vi "Refresh ECUs.vi"(8 "Type (Input)":T1, 9 "Frame Index":u32, 10 "ECU Name":string, 11 "ECUs":T2[](array[typedef])) -> (3 "ECUs out":T2[](array[typedef]))   [LabVIEW 2020, in "Communication Bus Template System Explorer.lvlib" / "Implementation.lvlib"]
uses:
  Implementation.lvlib
  Types/ECU.ctl
  <vilib>/NI VeriStand/Custom Device API/Custom Device Channel Type.ctl
  <vilib>/NI VeriStand/Custom Device API/Custom Device API.lvlib
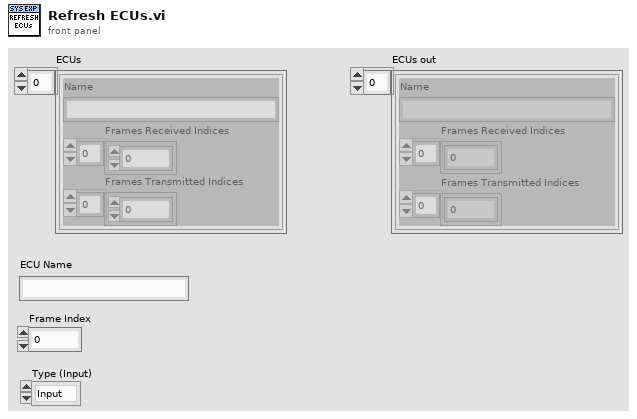
[diagram p1: front panel]
types:
  T1 = typedef "Custom Device API.lvlib/Custom Device Channel Type.ctl" = enum16{"Input", "Output"}
  T2 = typedef "Communication Bus Template System Explorer.lvlib/Implementation.lvlib/ECU.ctl" = cluster{"Name":string, "Frames Received Indices":u32[], "Frames Transmitted Indices":u32[]}
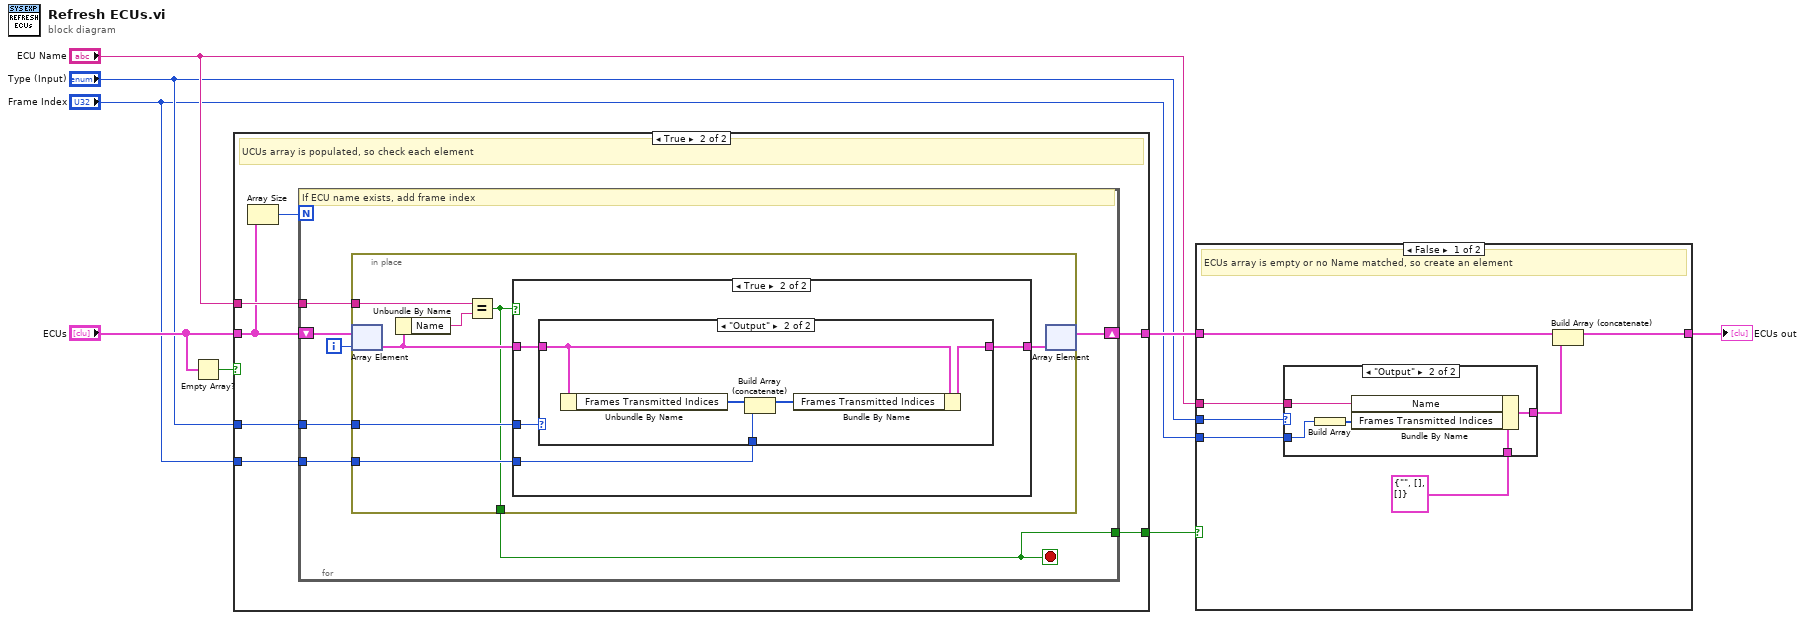
[diagram p0: block diagram]
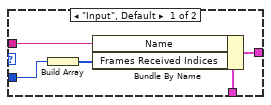
[diagram p2: hidden frame]
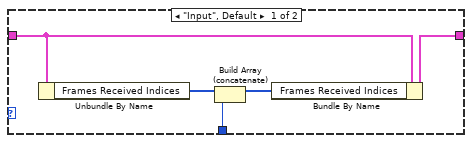
[diagram p6: hidden frame]
diagram:
  n1 = Empty Array?(array="ECUs") -> (empty?=w7:bool)
  n2 = case shown="True" w7 {
    selector: w7 -> [w9 _]
    tunnel: "ECU Name" -> [_ w17]
    tunnel: "Type (Input)" -> [_ w15]
    tunnel: "Frame Index" -> [_ w14]
    tunnel: [w10 w13] -> w5
    tunnel: "ECUs" -> [w10 w12]
    tunnel: [w9 w11] -> w6
    frame False {
      # "ECUs array is empty - need to create new element"
    }
    frame True {
      # "UCUs array is populated, so check each element"
      n3 = Array Size(array=w12) -> (size(s)=w16:i32)
      n4 = for {
        N: w16 -> [_]
        tunnel: w17 -> [w22]
        shift-right: [w19] -> w13
        shift-left: w12 -> [w24]
        tunnel: w15 -> [w21]
        tunnel: w14 -> [w20]
        tunnel: [w18] -> w11
        i -> [w23]
        stop <- w18 stop-if-true
        # "If ECU name exists, add frame index"
        n5 = in-place {
          in-place-border: w22 -> [w30]
          in-place-border: w21 -> [w28]
          in-place-border: w20 -> [w27]
          in-place-border: [w25] -> w18
          n6 = in-place-array #1(w24, w23) -> (w29:T2)
          n7 = Unbundle By Name(w29) -> ("Name"=w31:string)
          n8 = Equal?(x=w30, y=w31) -> (x = y?=w25:bool)
          n9 = case shown="True" w25 {
            tunnel: w29 -> [w32 w36]
            tunnel: w28 -> [_ w35]
            tunnel: w27 -> [_ w34]
            tunnel: [w32 w33] -> w26
            frame False {
            }
            frame True {
              n10 = case shown="\"Output\"" w35 {
                tunnel: w36 -> [w37 w42]
                tunnel: w34 -> [w40 w45]
                tunnel: [w38 w43] -> w33
                frame "Input", Default {
                  n11 = Unbundle By Name(w37) -> ("Frames Received Indices"=w41:u32[])
                  n12 = Build Array (concatenate)(w41, w40) -> (w39:u32[])
                  n13 = Bundle By Name(cluster=w37, "Frames Received Indices"=w39) -> (w38:T2)
                }
                frame "Output" {
                  n14 = Unbundle By Name(w42) -> ("Frames Transmitted Indices"=w46:u32[])
                  n15 = Build Array (concatenate)(w46, w45) -> (w44:u32[])
                  n16 = Bundle By Name(cluster=w42, "Frames Transmitted Indices"=w44) -> (w43:T2)
                }
              }
            }
          }
          n17 = in-place-array #1(w26) -> (w19:T2[])  [unwired: 1 out]
        }
      }
    }
  }
  n18 = case shown="False" w6 {
    tunnel: w5 -> [w48 w64]
    tunnel: [w53 w64] -> w4
    tunnel: "ECU Name" -> [w51 _]
    tunnel: "Type (Input)" -> [w50 _]
    tunnel: "Frame Index" -> [w49 _]
    frame False {
      # "ECUs array is empty or no Name matched, so create an element"
      n19 = case shown="\"Output\"" w50 {
        tunnel: T2 {"Name"="", "Frames Received Indices"=[], "Frames Transmitted Indices"=[]} ("ECU") -> [w58 w63]
        tunnel: w51 -> [w57 w62]
        tunnel: w49 -> [w56 w61]
        tunnel: [w54 w59] -> w47
        frame "Input", Default {
          n20 = Build Array(w56) -> (w55:u32[])
          n21 = Bundle By Name(cluster=w58, "Name"=w57, "Frames Received Indices"=w55) -> (w54:T2)
        }
        frame "Output" {
          n22 = Build Array(w61) -> (w60:u32[])
          n23 = Bundle By Name(cluster=w63, "Name"=w62, "Frames Transmitted Indices"=w60) -> (w59:T2)
        }
      }
      n24 = Build Array (concatenate)(w48, w47) -> (w53:T2[])
    }
    frame True {
      # "ECU name was previously found"
    }
  }
  "ECUs out" <- w4
